vi "读取LoggerSaveTime.vi"(8 "error in (no error)":errorcluster caption="错误输入（无错误）", 11 "Logger输入":refnum<class "Logger.lvclass">) -> (0 "error out":errorcluster caption="错误输出", 2 "LoggerSaveTime":T1, 3 "Logger输出":refnum<class "Logger.lvclass">)   [LabVIEW 2019, in "Logger.lvclass"]
uses:
  <userlib>/Logger/Logger.lvclass
  <userlib>/Logger/Ctls/LoggerSaveTime.ctl
  <userlib>/Logger/Logger.lvclass/Logger.ctl
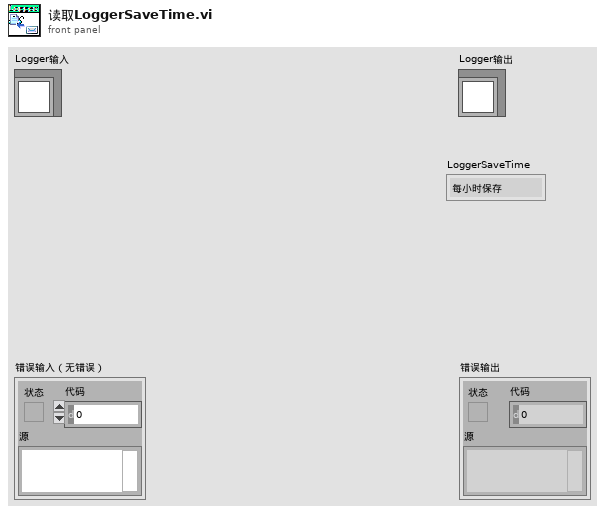
[diagram p1: front panel]
types:
  T1 = typedef "Logger.lvclass/LoggerSaveTime.ctl" = enum16{"每小时保存", "每天保存", "每周保存", "每月保存"}
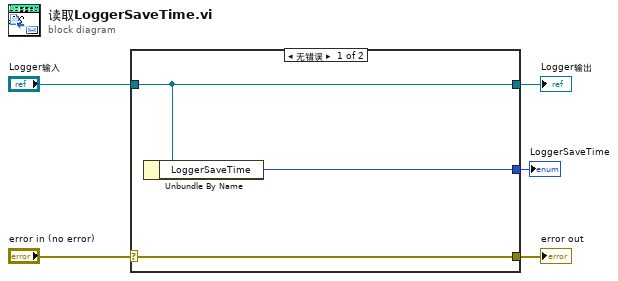
[diagram p0: block diagram]
diagram:
  n1 = case shown="无错误" "error in (no error)" {
    selector: "error in (no error)" -> [w8 w9]
    tunnel: [w8 w9] -> w4
    tunnel: [w7 w10] -> w2
    tunnel: "Logger输入" -> [w7 w10]
    tunnel: [w6 _] -> w1
    frame No Error {
      n2 = Unbundle By Name(w7) -> ("LoggerSaveTime"=w6:T1)
    }
    frame Error {
    }
  }
  "error out" <- w4
  "Logger输出" <- w2
  "LoggerSaveTime" <- w1
